vi "EnStateQueue.vi"(5 "Abort":bool, 7 "Pass?":bool, 8 "error in":errorcluster, 9 "States":T1 caption="NextState", 11 "QueueIn":variant) -> (0 "error out":errorcluster, 3 "QueueOut":variant)   [LabVIEW 2013]
uses:
  SysControl/States.ctl
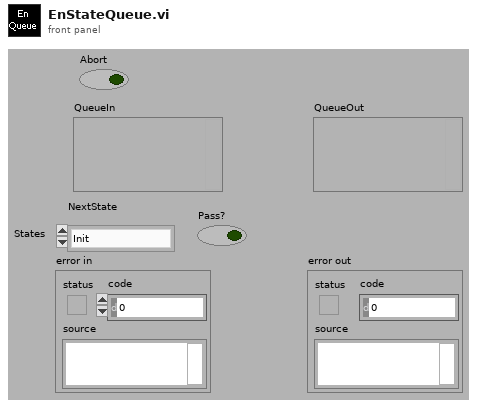
[diagram p1: front panel]
types:
  T1 = typedef "States.ctl" = enum16{"Init", "PreUUT", "Idle", "SetUp", "TestSequence", "PostUUT", "StopTest", "Debug Mode", "Selection Mode", "Loop Mode", "Error", "Wait"}
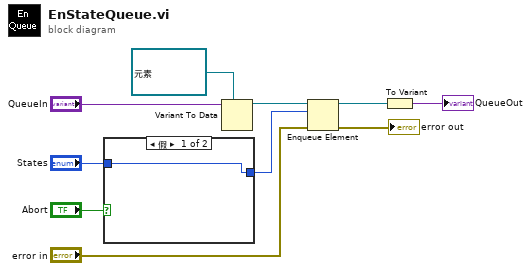
[diagram p0: block diagram]
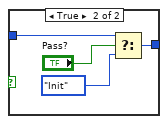
[diagram p2: hidden frame]
diagram:
  w6 = refnum<queue> refnum items=["Init", "PreUUT", "Idle", "SetUp", "TestSequence", "PostUUT", "StopTest", "Debug Mode", "Selection Mode", "Loop Mode", "Error", "Wait"] ("队列输出")
  n1 = case shown="假" "Abort" {
    tunnel: "States" -> [w11 w14]
    tunnel: [w11 w12] -> w4
    frame False {
    }
    frame True {
      n2 = Select(t=w14, s="Pass?", f=States."Init") -> (s? t:f=w12:T1)
    }
  }
  n3 = Variant To Data(type=w6, Variant="QueueIn") -> (data=w7:refnum<queue>)  [unwired: 1 in, 1 out]
  n4 = Enqueue Element(queue=w7, element=w4, error in (no error)="error in") -> (queue out=w8:refnum<queue>, error out=→"error out":errorcluster)  [unwired: 2 out]
  n5 = To Variant(anything=w8) -> (Variant=→"QueueOut":variant)
